vi "Vision Research Phantom Series PhCon PhFindCameraNumber.vi"(1 "pSerial":u32, 5 "Error In (no error)":errorcluster) -> (14 "CN out":u32=1, 19 "Error Out":errorcluster)   [LabVIEW 2013, in "VRI.lvlib"]
doc: "PhCon.dll\n\nPhFindCameraNumber\nHRESULT PhFindCameraNumber(UINT Serial, UINT *pCN);\n\nParameters Description\nSerial (in) Camera number.\npCN (out) Camera name maximum 15 char.\nReturn HRESULT (0=Ok)\nComments Scan all the connected cameras and find the camera that has\n the specified serial. Return the number of that camera in the\n pCN parameter if found or ERR_SerialNotFound if not.\n\nWritten by:\nBLOOMY CONTROLS, INC\nWINDSOR, CT 06095, USA\n860-298-9925\nwww.bloomy.com\nV1.0.0\nMay, 2004"
uses:
  VRI.lvlib
  Phantom DLLs/PhCon.dll
panel:
  # "For instructions on the use of this VI, press Ctrl+H to display the help window and move the mouse over the icon, controls, and indicators"
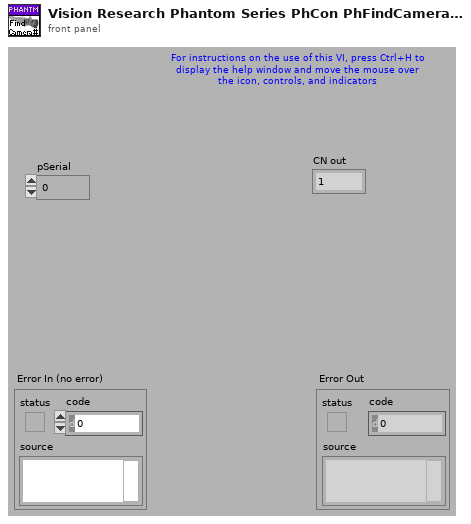
[diagram p1: front panel]
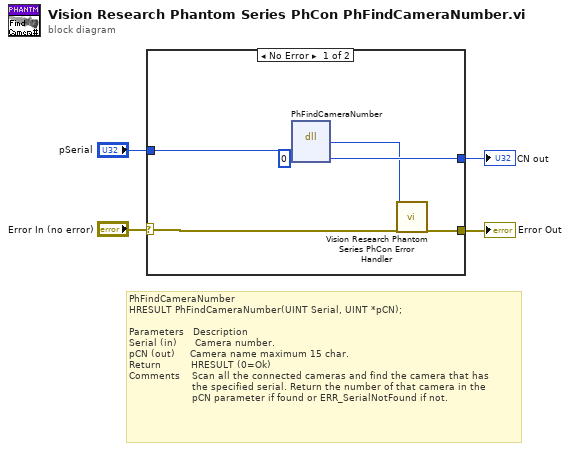
[diagram p0: block diagram]
diagram:
  # "PhFindCameraNumber\nHRESULT PhFindCameraNumber(UINT Serial, UINT *pCN);\n\nParameters   Description\nSerial (in)      Camera number.\npCN (out)     Camera name maximum 15 char.\nReturn          HRESULT (0=Ok)\nComments    Scan all the connected cameras and find the camera that has\n                     the specified serial. Return the number of that camera in the\n                     pCN parameter if found or ERR_SerialNotFound if not."
  n1 = case shown="No Error" "Error In (no error)" {
    selector: "Error In (no error)" -> [w10 w11]
    tunnel: [w9 w11] -> w3
    tunnel: "pSerial" -> [w8 _]
    tunnel: [w7 _] -> w1
    frame No Error {
      n2 = dll-call lib="C:/Projects/SDK/32-bit/Vision Research Phantom Series Labview Driver/Phantom DLLs/PhCon.dll" fn="PhFindCameraNumber"("pSerial"=w8, "pCN"=u32 0 ("pSerial")) -> ("HRESULT"=w6:i32, "pCN"=w7:u32)  [unwired: 4 in, 2 out]
      n3 = call "Vision Research Phantom Series PhCon Error Handler.vi"("ErrNo"=w6, "Error In (no error)"=w10) -> ("Error Out"=w9:errorcluster)  [unwired: 17 out]
    }
    frame Error {
    }
  }
  "Error Out" <- w3
  "CN out" <- w1
